vi "average_of_n_numbers.vi"(1 "Array":dbl[](array[numeric])) -> (0 "average of n numbers":dbl)   [LabVIEW 2020]
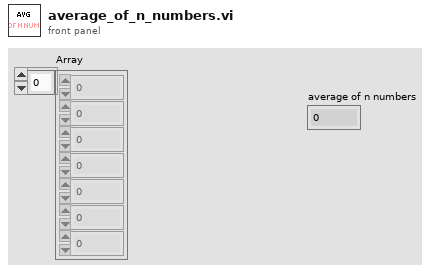
[diagram p1: front panel]
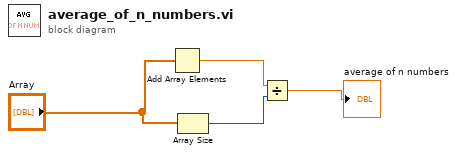
[diagram p0: block diagram]
diagram:
  n1 = Add Array Elements(numeric array="Array") -> (sum=w3:dbl)
  n2 = Array Size(array="Array") -> (size(s)=w2:i32)
  n3 = Divide(x=w3, y=w2) -> (x/y=→"average of n numbers":dbl)
